vi "jan29 sigma.vi"() -> ()   [LabVIEW 2014]
uses:
  <vilib>/Analysis/NI_AALBase.lvlib
panel:
  out "standard error of the mean":dbl
  out "Histogram":dynamicdata(graph)
  out "mean":dbl format="%0.2f"
  out "variance":dbl format="%0.2f"
  out "standard deviation":dbl format="%0.2f"
  out "sigma":dbl
  out "<i^2>":dbl
  out "most probable \nnumber of rolls, <i>":dbl
  out "sum of probabilities":dbl
  out "Waveform Graph":dbl[](graph)
  # "Analytical Calculations"
  # "Experimental Calculations"
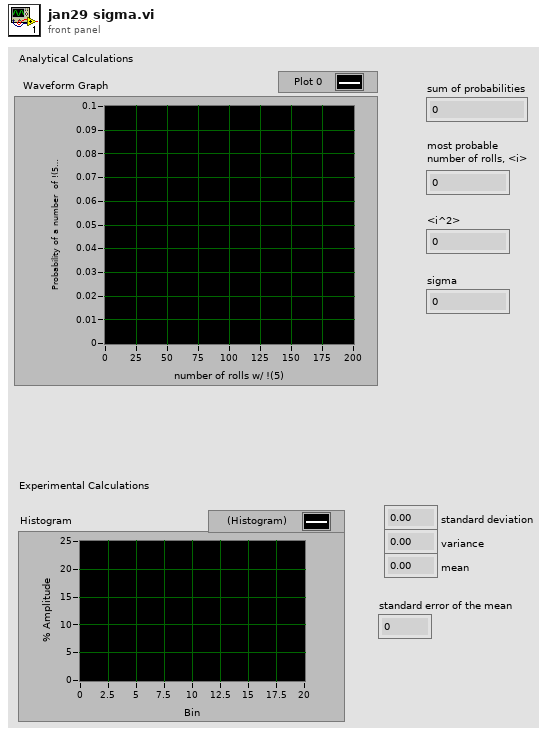
[diagram p1: front panel]
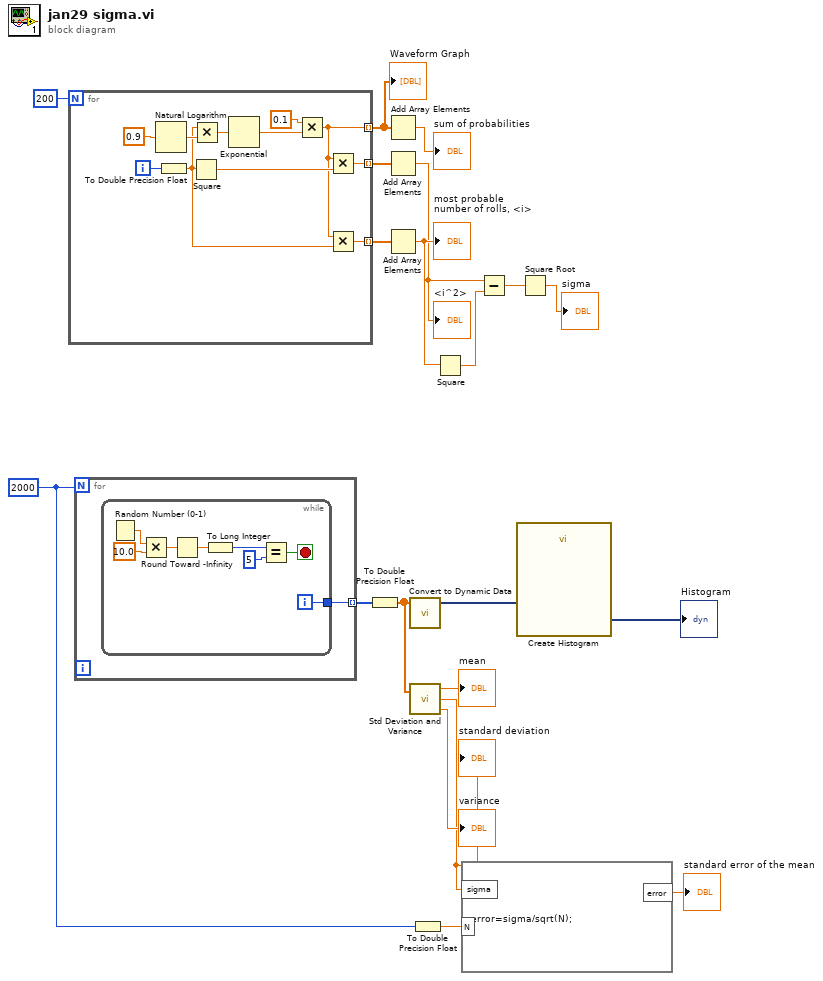
[diagram p0: block diagram]
diagram:
  w1 = 2000
  n1 = for {
    N: 200 -> [_]
    tunnel: [w22] -> w18 mode=indexing
    tunnel: [w25] -> w17 mode=indexing
    tunnel: [w21] -> w16 mode=indexing
    i -> [w28]
    n2 = Natural Logarithm(1:0.9 ("x")) -> (0:w29:dbl)
    n3 = To Double Precision Float(number=w28) -> (double precision float=w24:dbl)
    n4 = Square(x=w24) -> (x^2=w23:dbl)
    n5 = Multiply(x=w24, y=w29) -> (x*y=w27:dbl)
    n6 = Exponential(1:w27) -> (0:w26:dbl)
    n7 = Multiply(x=0.1, y=w26) -> (x*y=w22:dbl)
    n8 = Multiply(x=w22, y=w23) -> (x*y=w21:dbl)
    n9 = Multiply(x=w22, y=w24) -> (x*y=w25:dbl)
  }
  "Waveform Graph" <- w18
  n10 = for {
    N: w1 -> [_]
    tunnel: [w32] -> w10 mode=indexing
    n11 = while {
      tunnel: [w33] -> w32
      i -> [w33]
      stop <- w34 stop-if-true
      n12 = Random Number (0-1)() -> (number: 0 to 1=w40:dbl)
      n13 = Multiply(x=w40, y=10.0) -> (x*y=w38:dbl)
      n14 = Round Toward -Infinity(1:w38) -> (0:w37:dbl)
      n15 = To Long Integer(number=w37) -> (32bit integer=w36:i32)
      n16 = Equal?(x=w36, y=5) -> (x = y?=w34:bool)
    }
  }
  n17 = To Double Precision Float(number=w10) -> (double precision float=w7:dbl[])
  n18 = Add Array Elements(numeric array=w18) -> (sum=→"sum of probabilities":dbl)
  n19 = Add Array Elements(numeric array=w16) -> (sum=w13:dbl)
  "<i^2>" <- w13
  n20 = Add Array Elements(numeric array=w17) -> (sum=w14:dbl)
  "most probable \nnumber of rolls, <i>" <- w14
  n21 = call "Convert to Dynamic Data"("Array"=w7) -> ("Dynamic Data Type"=w6:dynamicdata)  [unwired: 3 in]
  n22 = call <vilib>:"Std Deviation and Variance.vi"("X"=w7) -> ("mean"=→"mean":dbl, "standard deviation"=w4:dbl, "variance"=→"variance":dbl)  [unwired: 1 in]
  "standard deviation" <- w4
  n23 = To Double Precision Float(number=w1) -> (double precision float=w2:dbl)
  n24 = Square(x=w14) -> (x^2=w15:dbl)
  n25 = formula code="error=sigma/sqrt(N);"("sigma"=w4, "N"=w2) -> ("error"=→"standard error of the mean":dbl)
  n26 = Subtract(x=w13, y=w15) -> (x-y=w12:dbl)
  n27 = call "Create Histogram"("Signal"=w6) -> ("Histogram"=→"Histogram":dynamicdata)  [unwired: 9 in, 1 out]
  n28 = Square Root(x=w12) -> (sqrt(x)=→"sigma":dbl)
